vi "EOL Check Motor Low Current Detection.vi"(6 "Error Table In":string[][](array[string]), 9 "Current Motion":T2=enum."Glass Slide Open", 10 "Current Data":sgl[][](array[numeric]), 11 "Motor Type":T1) -> (3 "Pass? Out":bool, 4 "Error Table Out":string[][](array[string]))   [LabVIEW 2018]
uses:
  02.Type Def's/All Motions.ctl
  05.UserVI's/type defs/EOL Motor Type.ctl
panel:
  out "Waveform Graph":sgl[](graph)
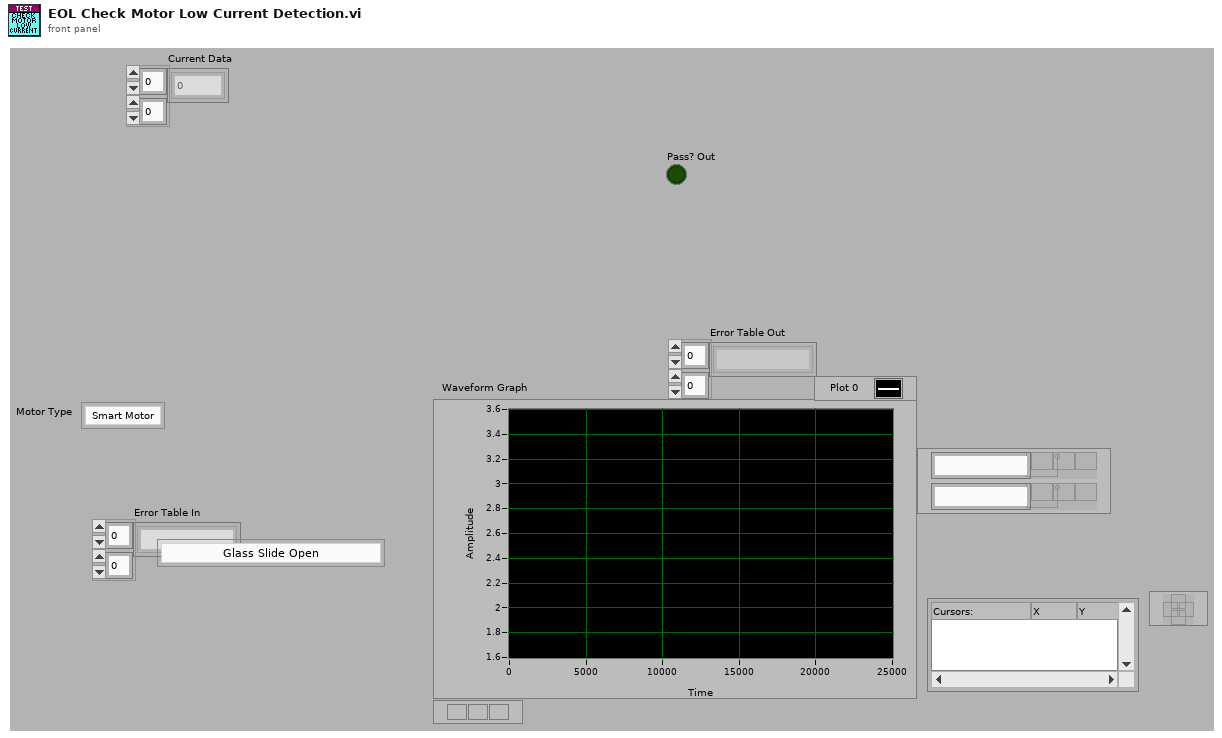
[diagram p1: front panel]
types:
  T1 = typedef "EOL Motor Type.ctl" = enum16{"Smart Motor", "Sensor Motor"}
  T2 = typedef "All Motions.ctl" = enum16{"Glass Teach", "Glass Slide Open", "Glass Slide Close", "Glass Vent Open", "Glass Vent Close", "Sunshade Teach", "Sunshade Open", "Sunshade Close", "Idle", "Sunshade Open 2", "Sunshade Close 2", "Glass Slide Open Sunshade Open", "Glass Slide Open Sunshade Close", "Glass Slide Close Sunshade Open", "Glass Slide Close Sunshade Close", "Glass Vent Open Sunshade Open", "Glass Vent Open Sunshade Close", "Glass Vent Close Sunshade Open", "Glass Vent Close Sunshade Close", "Express Glass Slide Open", "Express Glass Slide Close", "Express Glass Vent Open", "Express Glass Vent Close", "Express Sunshade Open", "Express Sunshade Close", "Express Sunshade Open 2", "Express Sunshade Close 2", "Express Glass Slide Open Sunshade Open", "Express Glass Slide Open Sunshade Close", "Express Glass Slide Close Sunshade Open", "Express Glass Slide Close Sunshade Close", "Express Glass Vent Open Sunshade Open", "Express Glass Vent Open Sunshade Close", "Express Glass Vent Close Sunshade Open", "Express Glass Vent Close Sunshade Close", "Goto Position Glass", "Goto Position Sunshade", "Sunshade Teach 2"}
  T3 = cluster{"Processed Current Data":sgl[], "Error Table In":string[][], "Pass?":bool, "Current Motion":T2, "Motor Type":T1}
  T4 = typedef "EOL Analog Input Control.ctl" = enum16{"SW PS  Volage", "Switch A", "Switch B", "Switch C", "Motor Voltage", "Motor Current", "ATS"}
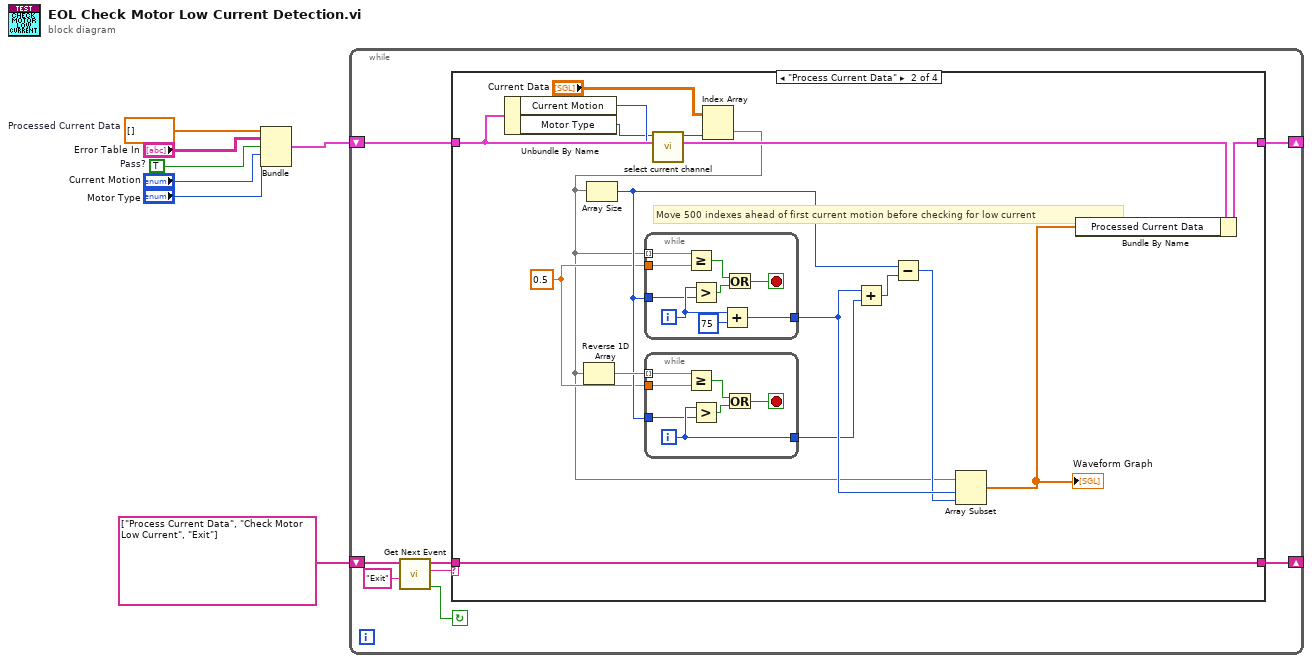
[diagram p0: block diagram]
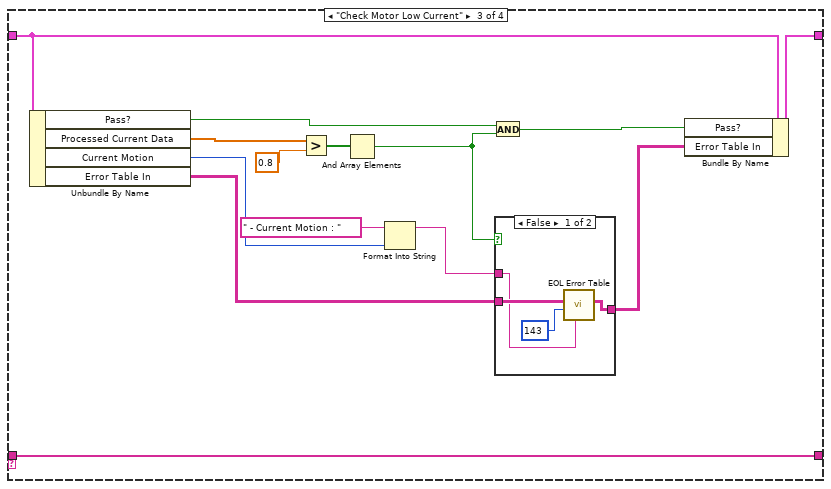
[diagram p3: hidden frame]
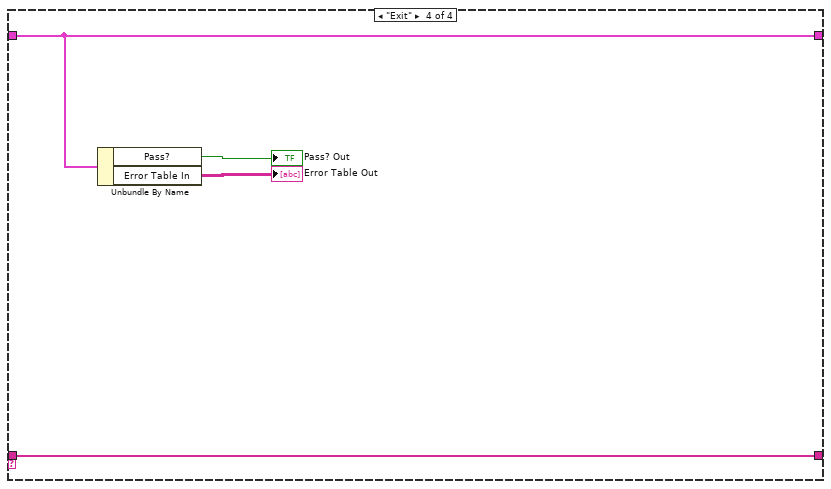
[diagram p5: hidden frame]
diagram:
  w2 = sgl[] []  # Processed Current Data
  w4 = TRUE  # Pass?
  n1 = Bundle("Processed Current Data"=w2, "Error Table In"="Error Table In", "Pass?"=w4, "Current Motion"="Current Motion", "Motor Type"="Motor Type") -> (w6:T3)  [unwired: 1 in]
  n2 = while {
    shift-right: [w13] -> _
    shift-left: string[] ["Process Current Data", "Check Motor Low Current", "Exit"] ("event queue out") -> [w12]
    shift-right: [w8] -> _
    shift-left: w6 -> [w9]
    stop <- w10 continue-if-true
    n3 = call "Get Next Event.vi"("Exit Event"="Exit", "event queue in"=w12) -> ("Condition (Exit:F)"=w10:bool, "next event"=w15:string, "event queue out"=w14:string[])  [unwired: 3 in]
    n4 = case shown="\"Process Current Data\"" w15 {
      tunnel: w14 -> [w17 w33 w63 w72]
      tunnel: [w17 w33 w63 w72] -> w13
      tunnel: w9 -> [w16 w23 w59 w69]
      tunnel: [w16 w26 w55 w69] -> w8
      frame "Error", Default {
      }
      frame "Process Current Data" {
        w24 = sgl 0.5 ("y")
        # "Move 500 indexes ahead of first current motion before checking for low current"
        n5 = Unbundle By Name(w23) -> ("Current Motion"=w21:T2, "Motor Type"=w20:T1)
        n6 = call "select current channel.vi"("Current Motion"=w21, "Motor Type"=w20) -> ("Analog channel"=w22:T4)  [unwired: 9 in]
        n7 = Index Array(array="Current Data", index (col)=w22) -> (element=w18:sgl[])  [unwired: 1 in]
        n8 = Reverse 1D Array(array=w18) -> (reversed array=w29:sgl[])
        n9 = Array Size(array=w18) -> (size(s)=w28:i32)
        n10 = while {
          tunnel: w18 -> [w49] mode=indexing
          tunnel: [w43] -> w31
          tunnel: w28 -> [w47]
          tunnel: w24 -> [w41]
          i -> [w48]
          stop <- w44 stop-if-true
          n11 = Greater Or Equal?(x=w49, y=w41) -> (x >= y?=w45:bool)
          n12 = Greater?(x=w48, y=w47) -> (0:w46:bool)
          n13 = Add(x=w48, y=75) -> (x+y=w43:i32)
          n14 = Or(x=w45, y=w46) -> (x .or. y?=w44:bool)
        }
        n15 = while {
          tunnel: w29 -> [w40] mode=indexing
          tunnel: [w39] -> w27
          tunnel: w28 -> [w38]
          tunnel: w24 -> [w34]
          i -> [w39]
          stop <- w35 stop-if-true
          n16 = Greater Or Equal?(x=w40, y=w34) -> (x >= y?=w36:bool)
          n17 = Greater?(x=w39, y=w38) -> (0:w37:bool)
          n18 = Or(x=w36, y=w37) -> (x .or. y?=w35:bool)
        }
        n19 = Add(x=w31, y=w27) -> (x+y=w32:i32)
        n20 = Subtract(x=w28, y=w32) -> (x-y=w30:i32)
        n21 = Array Subset(array=w18, index=w31, length=w30) -> (w25:sgl[])
        "Waveform Graph" <- w25
        n22 = Bundle By Name(cluster=w23, "Processed Current Data"=w25) -> (w26:T3)
      }
      frame "Check Motor Low Current" {
        n23 = Unbundle By Name(w59) -> ("Pass?"=w60:bool, "Processed Current Data"=w61:sgl[], "Current Motion"=w56:T2, "Error Table In"=w50:string[][])
        n24 = Greater?(x=w61, y=0.8) -> (0:w53:bool[])
        n25 = And Array Elements(Boolean array=w53) -> (logical AND=w52:bool)
        n26 = Format Into String(initial string=" - Current Motion : ", w56) -> (resulting string=w51:string)  [unwired: 2 in, 1 out]
        n27 = And(x=w60, y=w52) -> (x .and. y?=w57:bool)
        n28 = case shown="False" w52 {
          tunnel: w50 -> [w67 w68]
          tunnel: w51 -> [w66 _]
          tunnel: [w65 w68] -> w58
          frame False {
            n29 = call "EOL Error Table.vi"("Error Description"=w66, "Error No."=143, "Error Table In"=w67) -> ("Error Table Out"=w65:string[][])  [unwired: 7 in, 1 out]
          }
          frame True {
          }
        }
        n30 = Bundle By Name(cluster=w59, "Pass?"=w57, "Error Table In"=w58) -> (w55:T3)
      }
      frame "Exit" {
        n31 = Unbundle By Name(w69) -> ("Pass?"=→"Pass? Out":bool, "Error Table In"=→"Error Table Out":string[][])
      }
    }
  }
